vi "A33OutputOnOff_py.vi"(4 "Output mode (F:NORM,T:GATED)":bool, 5 "Enable Output (T: Enable)":bool=TRUE, 7 "Polarity (0: Normal)":i32(ring) items=["Normal", "Inverted"], 9 "Impedance (50.0 Ohms)":dbl=50.0, 10 "Channel (1: Channel1)":i32(ring)=1 items=["Channel1"=1, "Channel2"=2]) -> ()   [LabVIEW 2022 SP3]
doc: "Configures the output impedance and source impedance for the channel you specify."
uses:
  <vilib>/addons/zeromq/zmq_socket.lvclass
panel:
  out "Standalone":bool
  out "socket out":refnum<class "zmq_socket.lvclass">
  in  "socket in":refnum<class "zmq_socket.lvclass">
  out "error out":errorcluster
  out "resulting string":string
  in  "Instrument":string="AG33600A_Gen1"
  in  "error in (no error)":errorcluster
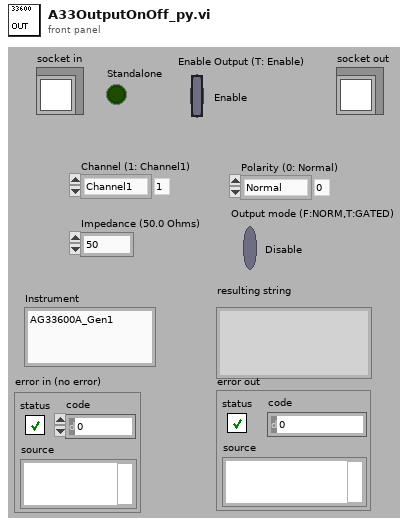
[diagram p1: front panel]
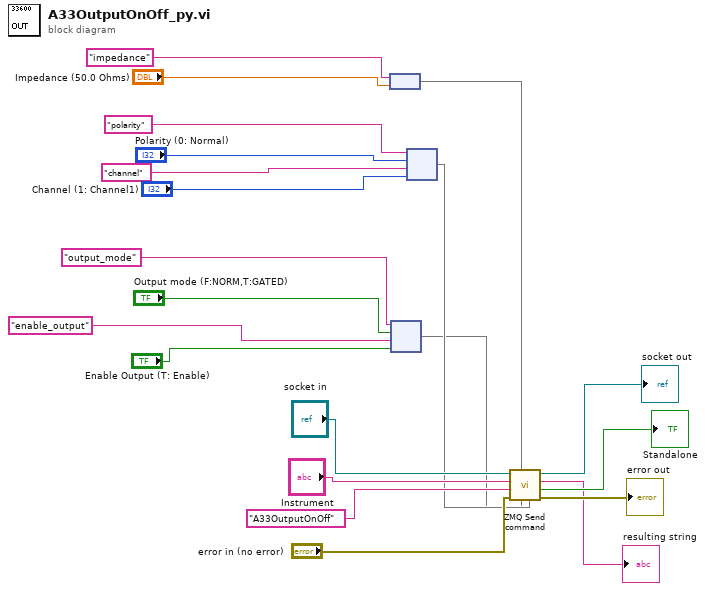
[diagram p0: block diagram]
diagram:
  n1 = node("impedance" ("key"), "Impedance (50.0 Ohms)") -> (w3:map{string, dbl})
  n2 = node("output_mode" ("key"), "Output mode (F:NORM,T:GATED)", "enable_output" ("key"), "Enable Output (T: Enable)") -> (w1:map{string, bool})
  n3 = node("polarity" ("key"), "Polarity (0: Normal)", "channel" ("key"), "Channel (1: Channel1)") -> (w2:map{string, i32})
  n4 = call "ZMQ Send command.vi"("Int args"=w2, "Bool args"=w1, "DBL args"=w3, "error in"="error in (no error)", "Command"="A33OutputOnOff", "Instrument"="Instrument", "socket in"="socket in") -> ("error out"=→"error out":errorcluster, "Standalone"=→"Standalone":bool, "Recieved message"=→"resulting string":string, "socket out"=→"socket out":refnum<class "zmq_socket.lvclass">)  [unwired: 1 in]
